vi "WriteRightData.vi"(8 "error in (no error)":errorcluster, 10 "Panel":T1, 11 "MAUI in":refnum<class "MAUI.lvclass">) -> (0 "error out":errorcluster, 3 "MAUI out":refnum<class "MAUI.lvclass">)   [LabVIEW 2016, in "MAUI.lvclass"]
uses:
  MAUI.lvclass
  Typedefs/PanelData.ctl
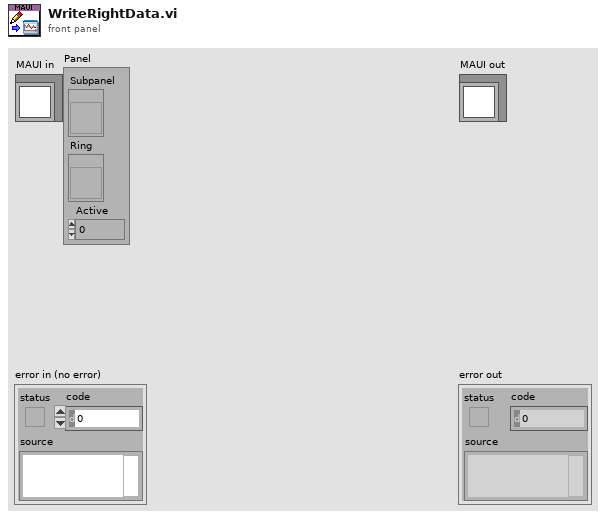
[diagram p1: front panel]
types:
  T1 = typedef "MAUI.lvclass/PanelData.ctl" = cluster{"Subpanel":refnum<vi>, "Ring":refnum<vi>, "Active":i32}
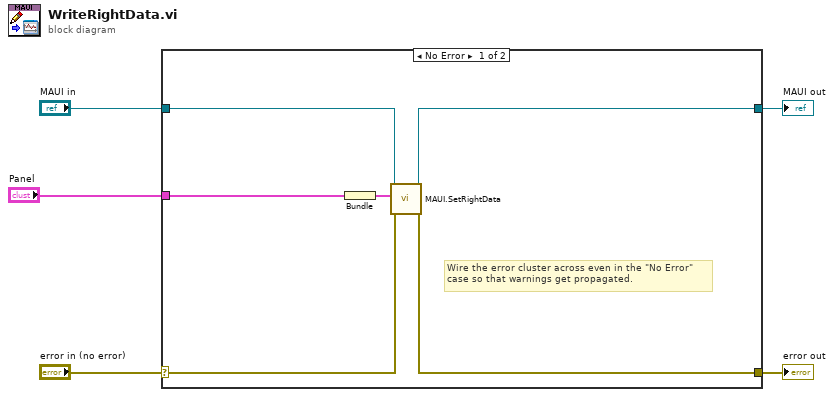
[diagram p0: block diagram]
diagram:
  n1 = case shown="No Error" "error in (no error)" {
    selector: "error in (no error)" -> [w9 w13]
    tunnel: [w8 w13] -> w4
    tunnel: [w7 w12] -> w2
    tunnel: "MAUI in" -> [w6 w12]
    tunnel: "Panel" -> [w10 _]
    frame No Error {
      # "Wire the error cluster across even in the \"No Error\"\ncase so that warnings get propagated."
      n2 = Bundle("Panel"=w10) -> (w11:cluster{"Panel":T1})  [unwired: 1 in]
      n3 = call "MAUI.SetRightData.vi"("error in (no error)"=w9, "SetRightData"=w11, "MAUI"=w6) -> ("error out"=w8:errorcluster, "MAUI out"=w7:refnum<class "MAUI.lvclass">)  [unwired: 7 in]
    }
    frame Error {
    }
  }
  "error out" <- w4
  "MAUI out" <- w2
